vi "Example Callback.vi"() -> ()   [LabVIEW 2010]
uses:
  C:/tf/play/labview/Tinkerforge.dll
  Tinkerforge.dll
panel:
  out "state":string
  in  "stop":bool
  in  "uid":string="XYZ"
  in  "port":i32=4223
  in  "host":string="localhost"
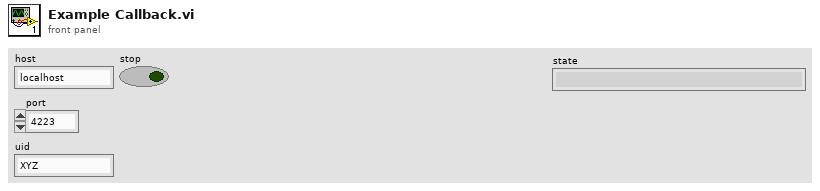
[diagram p1: front panel]
types:
  T1 = cluster{"buttonL":u8, "buttonR":u8, "ledL":u8, "ledR":u8}
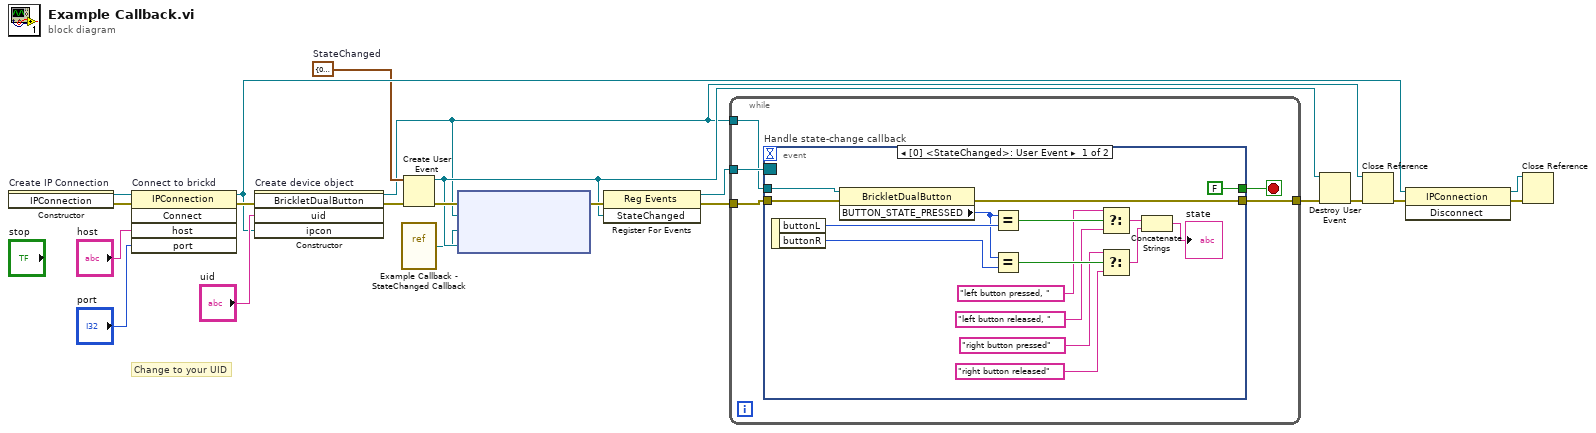
[diagram p0: block diagram]
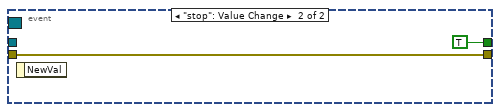
[diagram p2: hidden frame]
diagram:
  w5 = T1 {"buttonL"=0, "buttonR"=0, "ledL"=0, "ledR"=0}  # StateChanged
  # "Change to your UID"
  n1 = constructor on="Create IP Connection" class="IPConnection"() -> (reference out=w21:refnum<k24>, error out=w4:errorcluster)  [unwired: 3 in, 1 out]
  n2 = invoke on="Connect to brickd" class="IPConnection" method="Connect"(reference=w21, error in=w4, "host"="host", "port"="port") -> (reference out=w14:refnum<k24>, error out=w17:errorcluster)  [unwired: 1 in, 3 out]
  n3 = constructor on="Create device object" class="BrickletDualButton"(error in=w17, "uid"="uid", "ipcon"=w14) -> (reference out=w1:refnum<k24>, error out=w3:errorcluster)  [unwired: 2 in, 3 out]
  n4 = vi-ref "Example Callback - StateChanged Callback.vi"() -> ("vi reference"=w2:refnum<vi>)
  n5 = Create User Event(user event datatype=w5, error in=w3) -> (user event=w7:refnum<user-event>, error out=w12:errorcluster)
  n6 = node ("Register Event Callback")(w12, w1, w2, w7) -> (w11:errorcluster)  [unwired: 1 in, 1 out]
  n7 = register-events(error in=w11, w7) -> (reference out=w10:refnum<event-registration>, error out=w8:errorcluster)  [unwired: 1 in]
  n8 = while {
    tunnel: w10 -> [w26]
    tunnel: [w25] -> w9
    tunnel: w8 -> [w24]
    tunnel: w1 -> [w22]
    stop <- w23 stop-if-true
    n9 = event "Handle state-change callback" shown="[0] <StateChanged>: User Event" {
      selector: w26 -> [_ _]
      dyn-events: _ -> [_ _]
      timeout: _ -> [_ _]
      tunnel: [w39 w43] -> w25
      tunnel: w24 -> [w41 w43]
      tunnel: [FALSE TRUE] -> w23
      tunnel: w22 -> [w40 _]
      event User Event {
        n10 = event-data() -> ("buttonL"=w37:u8, "buttonR"=w38:u8)  [unwired: 1 in]
        n11 = property class="BrickletDualButton"(reference=w40, error in=w41) -> (error out=w39:errorcluster, "BUTTON_STATE_PRESSED"=w36:u8)  [unwired: 1 out]
        n12 = Equal?(x=w36, y=w37) -> (x = y?=w34:bool)
        n13 = Equal?(x=w36, y=w38) -> (x = y?=w35:bool)
        n14 = Select(t="left button pressed, ", s=w34, f="left button released, ") -> (s? t:f=w29:string)
        n15 = Select(t="right button pressed", s=w35, f="right button released") -> (s? t:f=w28:string)
        n16 = Concatenate Strings(w29, w28) -> (→"state":string)
      }
      event "stop": Value Change {
        n17 = event-data() -> ()  [unwired: 1 in, 1 out]
      }
    }
  }
  n18 = Destroy User Event(user event=w7, error in=w9) -> (error out=w6:errorcluster)
  n19 = Close Reference(reference=w1, error in (no error)=w6) -> (error out=w16:errorcluster)
  n20 = invoke class="IPConnection" method="Disconnect"(reference=w14, error in=w16) -> (reference out=w13:refnum<k24>, error out=w15:errorcluster)  [unwired: 1 in, 1 out]
  n21 = Close Reference(reference=w13, error in (no error)=w15) -> ()  [unwired: 1 out]
